vi "Request Token.vi"(6 "Callback URL":string="oob", 7 "Signature Method":T2=enum."HMAC-SHA1", 8 "error in (no error)":errorcluster, 9 "Consumer Secret":string, 10 "Consumer Key":string, 11 "Request URL":string) -> (0 "error out":errorcluster, 1 "OAuth Credentials (request)":T1={"Consumer Key"="", "Signature Method"=enum."HMAC-SHA1", "Token"="", "Version"="", "Token Secret"="", "Consumer Secret"=""}, 2 "Request Token (duplicate)":string)   [LabVIEW 2011, in "i3-oauth.lvlib"]
doc: "Obtains a request token for the application specified by the <B>Consumer Key</B> and <B>Consumer Secret</B>."
uses:
  i3-oauth.lvlib
  Controls/Signature Method.ctl
  Controls/OAuth Credentials.ctl
  Controls/HTTP Method.ctl
  <vilib>/httpClient/POSTBuffer.vi
  <vilib>/httpClient/LabVIEWHTTPClient.lvlib
panel:
  out "body":string
  out "headers":string
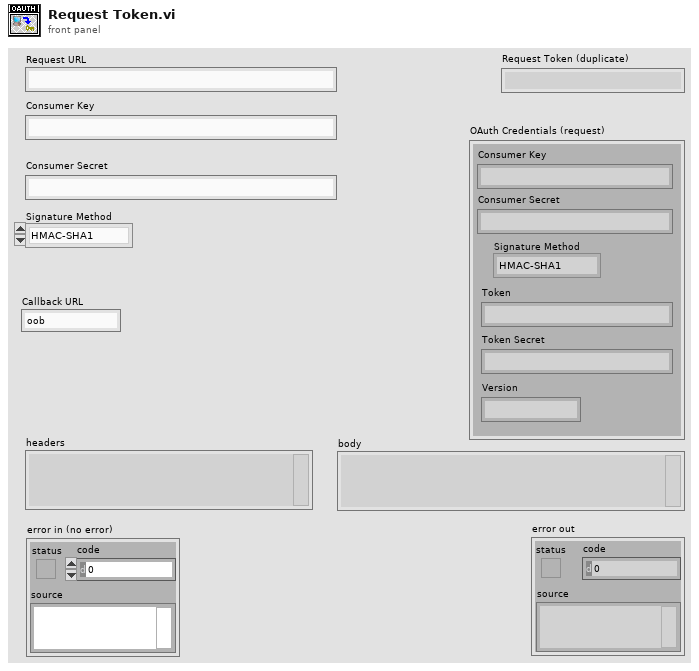
[diagram p1: front panel]
types:
  T1 = typedef "i3-oauth.lvlib/OAuth Credentials.ctl" = cluster{"Consumer Key":string, "Signature Method":T2, "Token":string, "Version":string, "Token Secret":string, "Consumer Secret":string}
  T2 = typedef "i3-oauth.lvlib/Signature Method.ctl" = enum16{"HMAC-MD5", "HMAC-SHA1", "HMAC-SHA224", "HMAC-SHA256", "HMAC-SHA384", "HMAC-SHA512"}
  T3 = typedef "i3-oauth.lvlib/HTTP Method.ctl" = enum16{"GET", "POST", "PUT", "DELETE"}
  T4 = typedef "i3-oauth.lvlib/key-value-pairs.ctl" = cluster{"key":string, "value":string}
  T5 = typedef "LabVIEWHTTPClient.lvlib/ClientHandle.ctl" = refnum<k1>
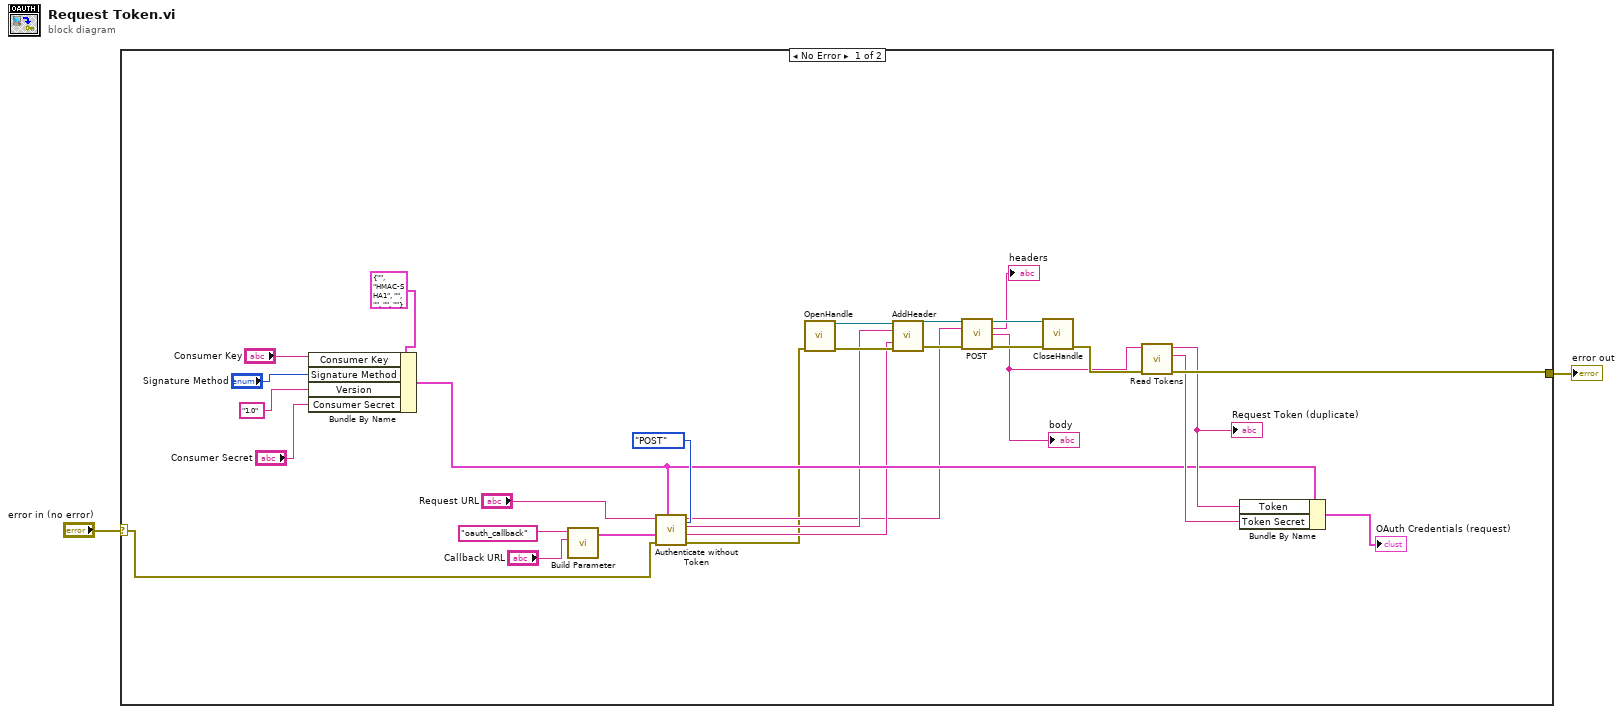
[diagram p0: block diagram]
diagram:
  n1 = case shown="No Error" "error in (no error)" {
    selector: "error in (no error)" -> [w3 w32]
    tunnel: [w24 w32] -> w1
    frame No Error {
      n2 = Bundle By Name(cluster=T1 {"Consumer Key"="", "Signature Method"=enum."HMAC-SHA1", "Token"="", "Version"="", "Token Secret"="", "Consumer Secret"=""} ("OAuth Credentials"), "Consumer Key"="Consumer Key", "Signature Method"="Signature Method", "Version"="1.0", "Consumer Secret"="Consumer Secret") -> (w8:T1)
      n3 = call "Build Parameter.vi"("Value"="Callback URL", "Key"="oauth_callback") -> ("Parameter Array"=w9:T4[])  [unwired: 9 in]
      n4 = call "Authenticate without Token.vi"("HTTP Method"=HTTP_Method."POST", "OAuth Credentials"=w8, "error in (no error)"=w3, "Header Parameters"=w9, "Base URL"="Request URL") -> ("error out"=w4:errorcluster, "Header Value"=w6:string, "Header Parameter"=w7:string, "Full URL"=w5:string)  [unwired: 2 in, 1 out]
      n5 = call <vilib>:"OpenHandle.vi"("error in (no error)"=w4) -> ("client handle out"=w31:T5, "error out"=w30:errorcluster)  [unwired: 13 in]
      n6 = call <vilib>:"AddHeader.vi"("client handle"=w31, "header"=w7, "value"=w6, "error in (no error)"=w30) -> ("client handle out"=w28:T5, "error out"=w29:errorcluster)  [unwired: 10 in]
      n7 = call-poly <vilib>:"POST.vi"("client handle"=w28, "url"=w5, "error in (no error)"=w29) -> ("client handle out"=w26:T5, "headers"=→"headers":string, "body"=w22:string, "error out"=w27:errorcluster)  [unwired: 9 in]
      "body" <- w22
      n8 = call <vilib>:"CloseHandle.vi"("client handle"=w26, "error in (no error)"=w27) -> ("error out"=w23:errorcluster)  [unwired: 13 in]
      n9 = call "Read Tokens.vi"("error in (no error)"=w23, "input string"=w22) -> ("error out"=w24:errorcluster, "Token Secret"=w20:string, "Token"=w21:string)  [unwired: 7 in]
      "Request Token (duplicate)" <- w21
      n10 = Bundle By Name(cluster=w8, "Token"=w21, "Token Secret"=w20) -> (→"OAuth Credentials (request)":T1)
    }
    frame Error {
    }
  }
  "error out" <- w1
